vi "fgv_ReferenceGlobal.vi"(8 "error in (no error)":errorcluster, 10 "Status":enum16{"Initialize", "Write", "Read"}(ring), 11 "ReferenceGlobal":T1={"RefDAQParam"={"Full Frame Size"=0, "Ref Field of View"=0.0, "Ref Zoom"=0, "Ref_dwellTime"=0.0, "Ref X-pixels-per-line(Npxr)"=0, "Ref Y-lines-per-image(Npyr)"=1, "Ref Z-lines-per-image"=5500, "Ignore Z lines"=0, "Ref Scan Cycles"=0, "Ref threshold XY"=4900, "Ref threshold Z"=0, "Ref average XY"=0, "Ref Average  Z"=0, "Proportional_scale"=0.0, "Integral_scale"=0.0, "Proportional_scale Z"=0.0, "Integral_scale Z"=1.0, "Diff_threshold"=1.0, "Diff_threshold _z"=0.0, "Sliding Average"=FALSE, "Ref count reset enabled"=FALSE}, "Reference Data"={"Refrence data path"=path "", "Reference Rectangle"=[], "AOL Z"=0.0, "No of pixels in a miniscan "=[], "Threshold"=[], "No of miniscans"=[], "Full Frame Size"=0, "Reference Image"=refnum, "dwelltime"=0.1, "Zoom"=1.0, "Field of View"=0.0, "Z Step"=1, "Z pixels"=1, "Z Lines"=1, "Z Ignore"=1, "Laser"=1}} {"RefDAQParam"."Proportional_scale Z" format="%#_15g"; "RefDAQParam"."Ref average XY" min=1 max=64 step=1; "RefDAQParam"."Diff_threshold" format="%#_15g"; "RefDAQParam"."Diff_threshold _z" format="%#_15g"; "RefDAQParam"."Proportional_scale" format="%#_15g"}) -> (0 "error out":errorcluster, 3 "ReferenceGlobal":T1={"RefDAQParam"={"Full Frame Size"=0, "Ref Field of View"=0.0, "Ref Zoom"=0, "Ref_dwellTime"=0.0, "Ref X-pixels-per-line(Npxr)"=0, "Ref Y-lines-per-image(Npyr)"=1, "Ref Z-lines-per-image"=5500, "Ignore Z lines"=0, "Ref Scan Cycles"=0, "Ref threshold XY"=4900, "Ref threshold Z"=0, "Ref average XY"=0, "Ref Average  Z"=0, "Proportional_scale"=0.0, "Integral_scale"=0.0, "Proportional_scale Z"=0.0, "Integral_scale Z"=1.0, "Diff_threshold"=1.0, "Diff_threshold _z"=0.0, "Sliding Average"=FALSE, "Ref count reset enabled"=FALSE}, "Reference Data"={"Refrence data path"=path "", "Reference Rectangle"=[], "AOL Z"=0.0, "No of pixels in a miniscan "=[], "Threshold"=[], "No of miniscans"=[], "Full Frame Size"=0, "Reference Image"=refnum, "dwelltime"=0.1, "Zoom"=1.0, "Field of View"=0.0, "Z Step"=1, "Z pixels"=1, "Z Lines"=1, "Z Ignore"=1, "Laser"=1}} {"RefDAQParam"."Proportional_scale Z" format="%#_15g"; "RefDAQParam"."Ref average XY" min=1 max=64 step=1; "RefDAQParam"."Diff_threshold" format="%#_15g"; "RefDAQParam"."Diff_threshold _z" format="%#_15g"; "RefDAQParam"."Proportional_scale" format="%#_15g"})   [LabVIEW 2020]
uses:
  <vilib>/vision/Image Controls.llb/IMAQ Image.ctl
  Typedefs/Reference_Globals.ctl
  Typedefs/ReferenceGlobal.ctl
  Acquisition/Typedefs/Ref DAQ Param.ctl
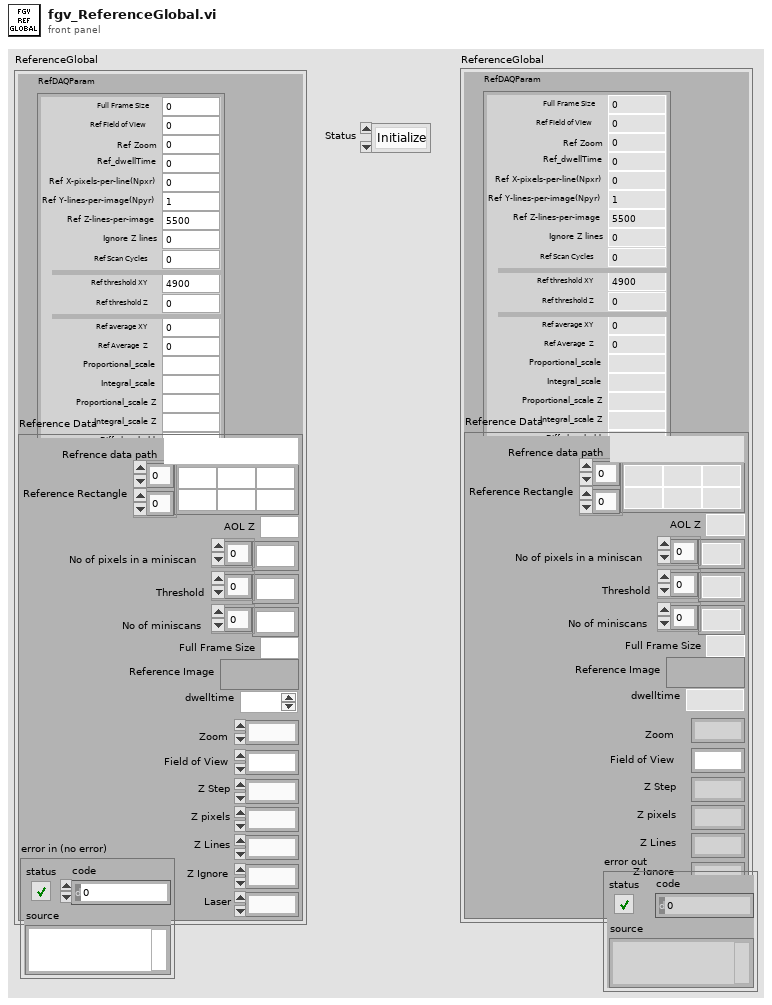
[diagram p1: front panel]
types:
  T1 = typedef "ReferenceGlobal.ctl" = cluster{"RefDAQParam":T2, "Reference Data":T3}
  T2 = typedef "Ref DAQ Param.ctl" = cluster{"Full Frame Size":u16, "Ref Field of View":sgl, "Ref Zoom":i8, "Ref_dwellTime":sgl, "Ref X-pixels-per-line(Npxr)":i16, "Ref Y-lines-per-image(Npyr)":i16, "Ref Z-lines-per-image":i16, "Ignore Z lines":i16, "Ref Scan Cycles":i32, "Ref threshold XY":u16, "Ref threshold Z":u16, "Ref average XY":u16, "Ref Average  Z":u16, "Proportional_scale":fxp<+,16,2>, "Integral_scale":fxp<+/-,16,12>, "Proportional_scale Z":fxp<+,16,2>, "Integral_scale Z":fxp<+/-,16,12>, "Diff_threshold":fxp<+,16,2>, "Diff_threshold _z":fxp<+,16,2>, "Sliding Average":bool, "Ref count reset enabled":bool}
  T3 = typedef "Reference_Globals.ctl" = cluster{"Refrence data path":path, "Reference Rectangle":i16[][], "AOL Z":dbl, "No of pixels in a miniscan ":i32[], "Threshold":i16[], "No of miniscans":i32[], "Full Frame Size":u16, "Reference Image":T4, "dwelltime":dbl, "Zoom":dbl, "Field of View":dbl, "Z Step":i8, "Z pixels":i32, "Z Lines":u8, "Z Ignore":u8, "Laser":u8}
  T4 = typedef "IMAQ Image.ctl" = refnum<image>
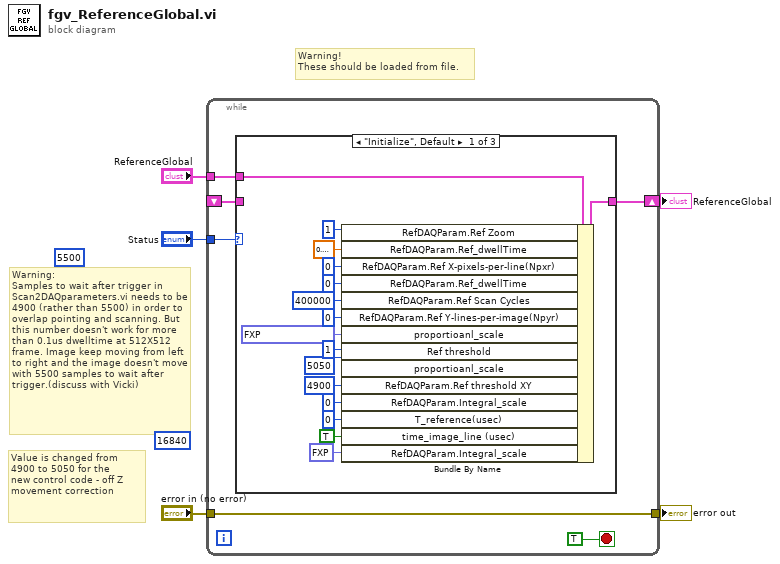
[diagram p0: block diagram]
diagram:
  (unwired) u16 5500 ("Samples Wait after Trigger")
  (unwired) u32 16840 ("Slip Cycle")
  # "Value is changed from 4900 to 5050 for the \nnew control code - off Z movement correction"
  # "Warning:\nSamples to wait after trigger in Scan2DAQparameters.vi needs to be 4900 (rather than 5500) in order to overlap pointing and scanning. But this number doesn't work for more than 0.1us dwelltime at 512X512 frame. Image keep moving from left to right and the image doesn't move with 5500 samples to wait after trigger.(discuss with Vicki)"
  # "Warning!\nThese should be loaded from file."
  n1 = while {
    tunnel: "Status" -> [w10]
    shift-right: [w9] -> w3
    shift-left: _ -> [w8]
    tunnel: "ReferenceGlobal" -> [w7]
    tunnel: "error in (no error)" -> [w6]
    tunnel: [w6] -> w1
    stop <- TRUE stop-if-true
    n2 = case shown="\"Initialize\", Default" w10 {
      tunnel: [w26 w28 w29] -> w9
      tunnel: w8 -> [_ _ w29]
      tunnel: w7 -> [w27 w28 _]
      frame "Initialize", Default {
        n3 = Bundle By Name(cluster=w27, "RefDAQParam.Ref Zoom"=i8 1 ("Ref Zoom"), "RefDAQParam.Ref_dwellTime"=sgl 0.1 ("Ref_dwellTime"), "RefDAQParam.Ref X-pixels-per-line(Npxr)"=i16 0 ("Ref X-pixels-per-line(Npxr)"), "RefDAQParam.Ref_dwellTime"=i16 0 ("Ref Y-pixels-per-line(NPyr)"), "RefDAQParam.Ref Scan Cycles"=400000 ("Ref Scan Cycles"), "RefDAQParam.Ref Y-lines-per-image(Npyr)"=u16 0 ("threshold"), "proportioanl_scale"=fxp<+,16,2> 1.5999755859375, "Ref threshold"=u16 1 ("Average"), "proportioanl_scale"=u16 5050 ("Samples Wait after Trigger"), "RefDAQParam.Ref threshold XY"=u16 4900 ("AOD fill"), "RefDAQParam.Integral_scale"=0 ("StartupDelay"), "T_reference(usec)"=u32 0 ("Slip Cycle"), "time_image_line (usec)"=TRUE ("Add Cycle"), "RefDAQParam.Integral_scale"=fxp<+/-,16,12> 450.0 ("Integral_scale")) -> (w26:T1)
      }
      frame "Write" {
      }
      frame "Read" {
      }
    }
  }
  "ReferenceGlobal" <- w3
  "error out" <- w1
